vi "Set System Time.vi"(8 "error in (no error)":errorcluster, 10 "Time:Current time":timestamp, 11 "session in":refnum<k21>="localhost") -> (0 "error out":errorcluster, 1 "Time After":timestamp, 2 "Time Before":timestamp, 3 "session out":refnum<k21>)   [LabVIEW 2012]
uses:
  <vilib>/nisyscfg/Find Hardware.vi
  <vilib>/nisyscfg/Save Changes (Hardware).vi
  <vilib>/nisyscfg/nisyscfg.lvlib
  <resource>/objmgr/nisysapi.rc
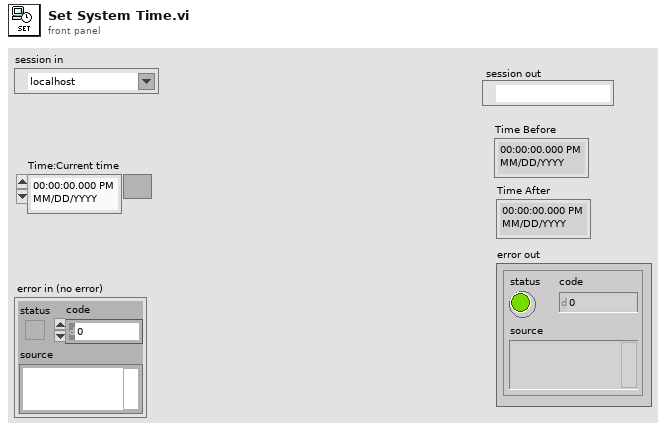
[diagram p1: front panel]
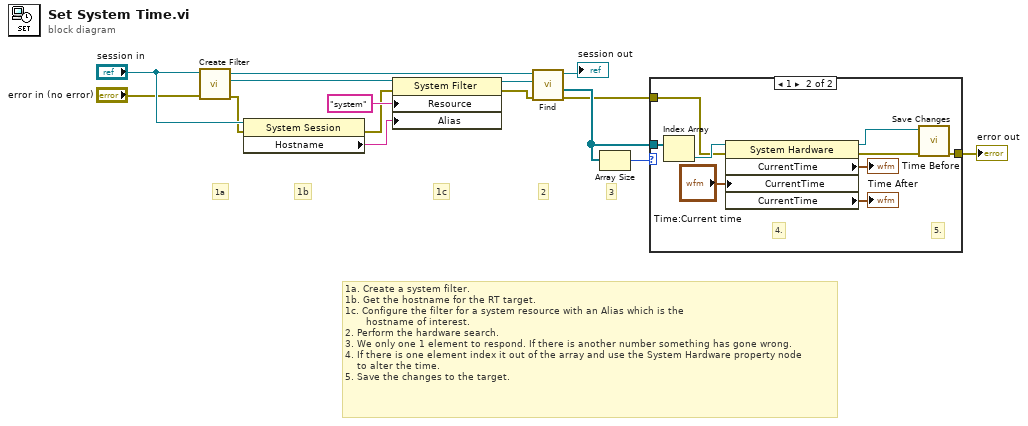
[diagram p0: block diagram]
diagram:
  # "1a. Create a system filter.\n1b. Get the hostname for the RT target.\n1c. Configure the filter for a system resource with an Alias which is the\n       hostname of interest.\n2. Perform the hardware search.\n3. We only one 1 element to respond. If there is another number something has gone wrong.\n4. If there is one element index it out of the array and use the System Hardware property node\n    to alter the time.\n5. Save the changes to the target."
  # "3"
  # "2"
  # "1c"
  # "1b"
  # "1a"
  n1 = call <vilib>:"Create Filter.vi"("error in (no error)"="error in (no error)", "session in"="session in") -> ("error out"=w8:errorcluster, "filter out"=w15:refnum<k20>, "session out"=w13:refnum<k21>)  [unwired: 7 in]
  n2 = property class="System Session"(reference="session in", error in=w8) -> (error out=w6:errorcluster, "Hostname"=w11:string)  [unwired: 1 out]
  n3 = property class="System Filter"(reference=w15, error in=w6, "Resource"="system" ("Expert Info:Resource Name"), "Alias"=w11) -> (reference out=w14:refnum<k20>, error out=w7:errorcluster)
  n4 = call-poly <vilib>:"Find.vi"("error in (no error)"=w7, "filter in"=w14, "session in"=w13) -> ("error out"=w3:errorcluster, "resources out"=w4:refnum<k20>[], "session out"=→"session out":refnum<k21>)  [unwired: 5 in, 1 out]
  n5 = Array Size(array=w4) -> (size(s)=w2:i32)
  n6 = case shown="1" w2 {
    tunnel: [w16 w20] -> w5
    tunnel: w4 -> [_ w19]
    tunnel: w3 -> [w16 w18]
    frame 0, Default {
    }
    frame 1 {
      # "5."
      # "4."
      n7 = Index Array(array=w19) -> (element=w25:refnum<k20>)  [unwired: 1 in]
      n8 = property class="System Hardware"(reference=w25, error in=w18, "CurrentTime"="Time:Current time") -> (reference out=w22:refnum<k20>, error out=w21:errorcluster, "CurrentTime"=→"Time Before":timestamp, "CurrentTime"=→"Time After":timestamp)
      n9 = call-poly <vilib>:"Save Changes.vi"("error in (no error)"=w21, "resource in"=w22) -> ("error out"=w20:errorcluster)  [unwired: 6 in, 3 out]
    }
  }
  "error out" <- w5
